vi "Main - CurrentTime (SubVI).vi"() -> (3 "Seconds":dbl format="%#.6f", 5 "Time":string)   [LabVIEW 2019]
uses:
  <vilib>/httpClient/LabVIEWHTTPClient.lvlib
  <vilib>/httpClient/POSTBuffer.vi
panel:
  in  "current time":timestamp
  out "body":string
  out "error out":errorcluster
  in  "error in (no error)":errorcluster
  # "1759204147"
  # "1759117720"
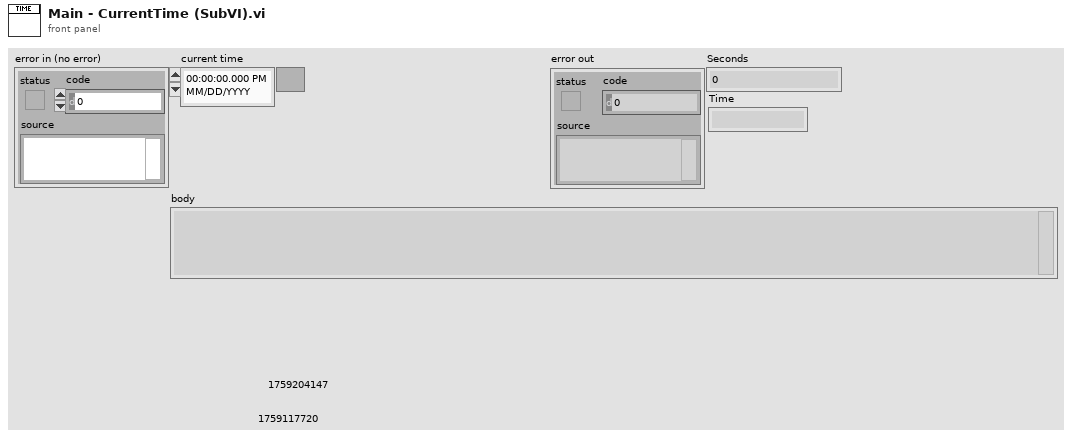
[diagram p1: front panel]
types:
  T1 = typedef "LabVIEWHTTPClient.lvlib/ClientHandle.ctl" = refnum<k1>
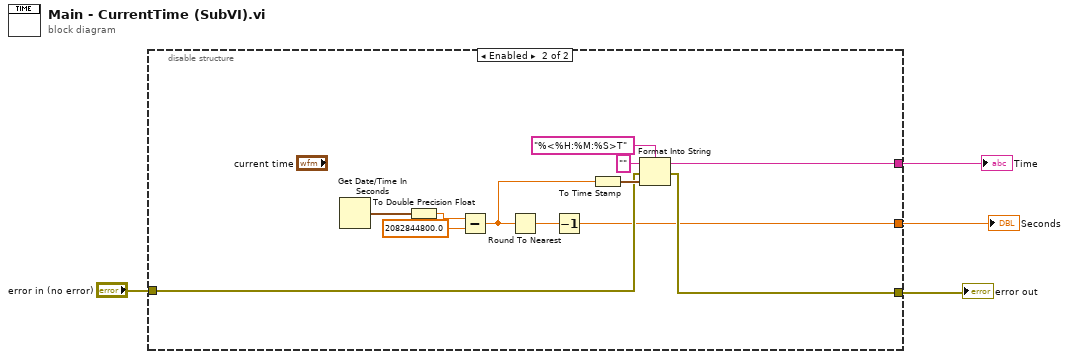
[diagram p0: block diagram]
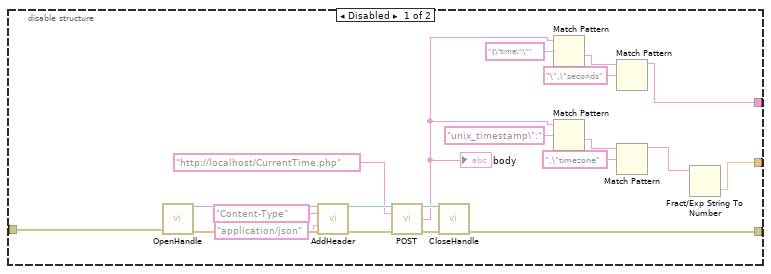
[diagram p2: hidden frame]
diagram:
  n1 = disable-structure shown="Enabled" {
    disable-tunnel: "error in (no error)" -> [w8 w30]
    disable-tunnel: [w7 w29] -> w3
    disable-tunnel: [w5 w28] -> w2
    disable-tunnel: [w6 w27] -> w1
    frame Disabled {
      n2 = call <vilib>:"OpenHandle.vi"("error in (no error)"=w8) -> ("client handle out"=w23:T1, "error out"=w25:errorcluster)  [unwired: 13 in]
      n3 = call <vilib>:"AddHeader.vi"("client handle"=w23, "header"="Content-Type", "value"="application/json", "error in (no error)"=w25) -> ("client handle out"=w22:T1, "error out"=w24:errorcluster)  [unwired: 10 in]
      n4 = call-poly <vilib>:"POST.vi"("client handle"=w22, "url"="http://localhost/CurrentTime.php", "error in (no error)"=w24) -> ("client handle out"=w17:T1, "body"=w9:string, "error out"=w18:errorcluster)  [unwired: 9 in, 1 out]
      "body" <- w9
      n5 = call <vilib>:"CloseHandle.vi"("client handle"=w17, "error in (no error)"=w18) -> ("error out"=w7:errorcluster)  [unwired: 13 in]
      n6 = Match Pattern(string=w9, regular expression="{\"time\":\"") -> (after substring=w11:string)  [unwired: 1 in, 3 out]
      n7 = Match Pattern(string=w9, regular expression="unix_timestamp\":") -> (after substring=w15:string)  [unwired: 1 in, 3 out]
      n8 = Match Pattern(string=w11, regular expression="\",\"seconds") -> (before substring=w5:string)  [unwired: 1 in, 3 out]
      n9 = Match Pattern(string=w15, regular expression=",\"timezone") -> (before substring=w13:string)  [unwired: 1 in, 3 out]
      n10 = Fract/Exp String To Number(string=w13) -> (number=w6:dbl)  [unwired: 3 in, 1 out]
    }
    frame Enabled {
      n11 = Get Date/Time In Seconds() -> (seconds since 1Jan1904=w26:timestamp)
      n12 = To Double Precision Float(number=w26) -> (double precision float=w34:dbl)
      n13 = Subtract(x=w34, y=2082844800.0) -> (x-y=w36:dbl)
      n14 = Round To Nearest(number=w36) -> (nearest integer value=w35:dbl)
      n15 = Decrement(x=w35) -> (x-1=w27:dbl)
      n16 = To Time Stamp(1:w36) -> (0:w37:timestamp)
      n17 = Format Into String(format string="%<%H:%M:%S>T", initial string="", error in=w30, w37) -> (resulting string=w28:string, error out=w29:errorcluster)
    }
  }
  "Seconds" <- w1
  "Time" <- w2
  "error out" <- w3
